vi "Logging with Helper-VIs.vi"() -> ()   [LabVIEW 2016]
doc: "HSE-Logger example using the helper VIs."
uses:
  HSE-Logger/LogLevel.ctl
  HSE-Logger/Formatter/HSE_v2_Formatter/HSE_v2_Formatter.lvclass
  C:/_work/hampel-soft/open-source/hse-logger/Source/HSE-Logger/Formatter/Formatter.lvclass
  HSE-Logger/Handler/UserEventHandler/UserEventHandler.lvclass
  C:/_work/hampel-soft/open-source/hse-logger/Source/HSE-Logger/Handler/Handler.lvclass
  HSE-Logger/Handler/FileHandler/FileHandler.lvclass
  HSE-Logger/hse-logger.lvlib
  HSE-Logger/Formatter/JSONLFormatter/JSONLFormatter.lvclass
  HSE-Logger/Formatter/Formatter.lvclass
panel:
  out "Displays log messages =>":string
  in  "btn_Log":bool
  in  "Level of Log Message":T1(ring)
  in  "Log Error":errorcluster
  in  "Log Message":string
  out "Display User Event Logs":string
  in  "btn_Exit":bool
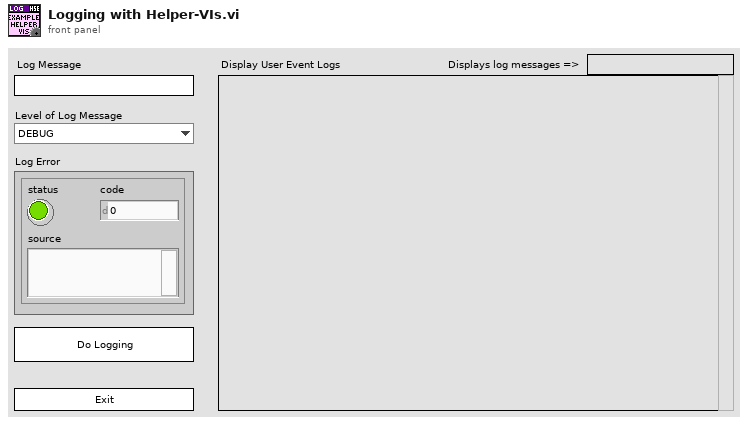
[diagram p1: front panel]
types:
  T1 = enum16{"DEBUG", "INFO", "WARNING", "ERROR", "CRITICAL"}
  T2 = typedef "hse-logger.lvlib/LogLevel.ctl" = enum16{"DEBUG", "INFO", "WARNING", "ERROR", "CRITICAL"}
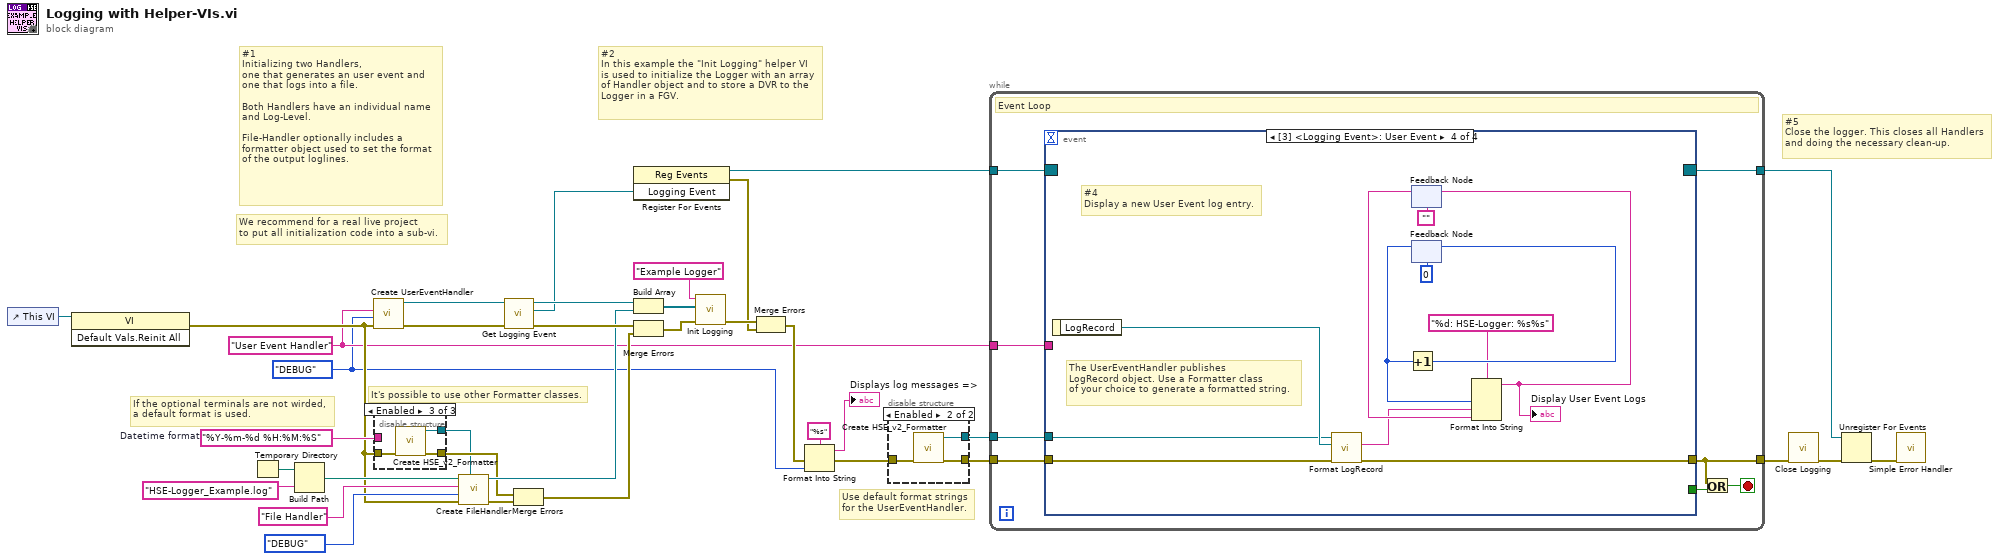
[diagram p0: block diagram]
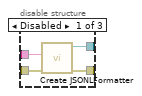
[diagram p2: hidden frame]
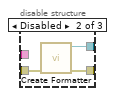
[diagram p3: hidden frame]
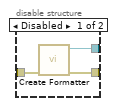
[diagram p4: hidden frame]
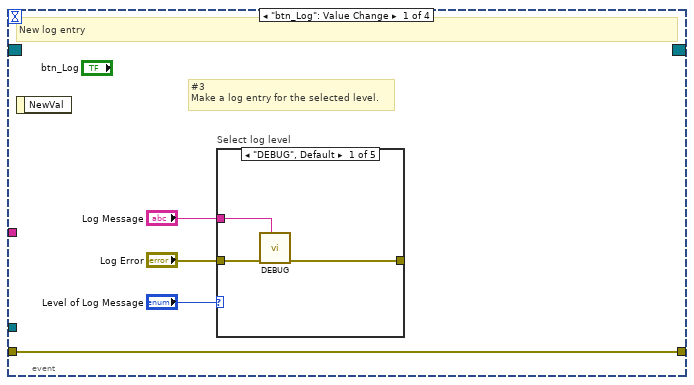
[diagram p5: hidden frame]
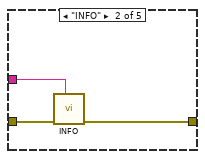
[diagram p6: hidden frame]
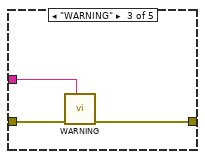
[diagram p7: hidden frame]
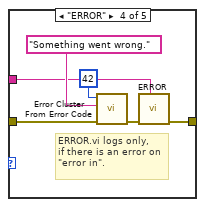
[diagram p8: hidden frame]
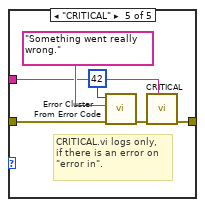
[diagram p9: hidden frame]
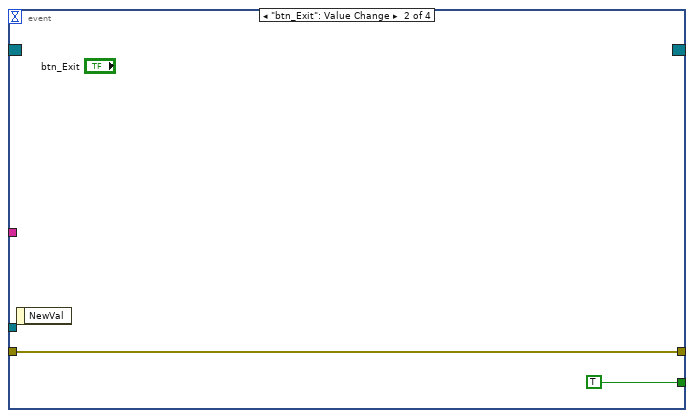
[diagram p10: hidden frame]
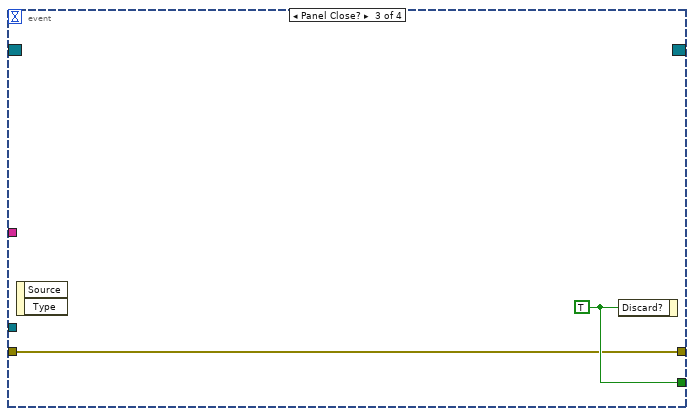
[diagram p11: hidden frame]
diagram:
  w9 = "%Y-%m-%d %H:%M:%S"  # Datetime format
  w1 = LogLevel."DEBUG" ("Level")
  w2 = "User Event Handler" ("Name")
  # "Use default format strings\nfor the UserEventHandler."
  # "If the optional terminals are not wirded,\na default format is used."
  # "It's possible to use other Formatter classes."
  # "We recommend for a real live project\nto put all initialization code into a sub-vi."
  # "#5\nClose the logger. This closes all Handlers\nand doing the necessary clean-up."
  # "#2\nIn this example the \"Init Logging\" helper VI \nis used to initialize the Logger with an array\nof Handler object and to store a DVR to the\nLogger in a FGV."
  # "#1\nInitializing two Handlers,\none that generates an user event and\none that logs into a file.\n\nBoth Handlers have an individual name\nand Log-Level.\n\nFile-Handler optionally includes a\nformatter object used to set the format\nof the output loglines."
  n1 = control-ref of="This VI"() -> (w25:refnum<vi>)
  n2 = invoke class="VI" method="Default Vals.Reinit All"(reference=w25) -> (error out=w8:errorcluster)  [unwired: 2 in, 2 out]
  n3 = Temporary Directory() -> (w24:path)
  n4 = Build Path(base path=w24, name or relative path="HSE-Logger_Example.log") -> (appended path=w14:path)
  n5 = call "Create UserEventHandler.vi"("error in"=w8, "Level"=w1, "Name"=w2) -> ("error out"=w17:errorcluster, "UserEventHandler out"=w13:refnum<class "UserEventHandler.lvclass">)  [unwired: 7 in]
  n6 = disable-structure shown="Enabled" {
    disable-tunnel: w9 -> [w40 _ _]
    disable-tunnel: w8 -> [w39 w43 w46]
    disable-tunnel: [w38 w42 w45] -> w7
    disable-tunnel: [w37 w41 w44] -> w3
    frame Disabled {
      n7 = call "Create JSONLFormatter.vi"("error in"=w39, "Datetime format"=w40) -> ("error out"=w38:errorcluster, "JSONLFormatter out"=w37:refnum<class "JSONLFormatter.lvclass">)  [unwired: 8 in]
    }
    frame Disabled {
      n8 = call "Create Formatter.vi"("error in"=w43) -> ("error out"=w42:errorcluster, "Formatter out"=w41:refnum<class "Formatter.lvclass">)  [unwired: 9 in]
    }
    frame Enabled {
      n9 = call "Create HSE_v2_Formatter.vi"("error in"=w46) -> ("error out"=w45:errorcluster, "HSE_v2_Formatter out"=w44:refnum<class "HSE_v2_Formatter.lvclass">)  [unwired: 9 in]
    }
  }
  n10 = call "Create FileHandler.vi"("Formatter.lvclass"=w3, "error in"=w8, "Level"=LogLevel."DEBUG", "Name"="File Handler", "Filepath"=w14) -> ("error out"=w12:errorcluster, "FileHandler out"=w10:refnum<class "FileHandler.lvclass">)  [unwired: 5 in]
  n11 = call-dynamic "Get Logging Event.vi"("error in"=w17, "UserEventHandler in"=w13) -> ("error out"=w33:errorcluster, "Logging Event"=w31:refnum<user-event>, "UserEventHandler out"=w32:refnum<class "UserEventHandler.lvclass">)  [unwired: 7 in]
  n12 = Merge Errors(w7, w12) -> (w11:errorcluster)
  n13 = register-events(w31) -> (reference out=w30:refnum<event-registration>, error out=w28:errorcluster)  [unwired: 2 in]
  n14 = Build Array(w32, w10) -> (w35:refnum<class "Handler.lvclass">[])
  n15 = Merge Errors(w33, w11) -> (w34:errorcluster)
  n16 = call "Init Logging.vi"("error in"=w34, "Handlers"=w35, "Name"="Example Logger") -> ("error out"=w29:errorcluster)  [unwired: 8 in]
  n17 = Merge Errors(w29, w28) -> (w21:errorcluster)
  n18 = Format Into String(format string="%s", error in=w21, w1) -> (resulting string=→"Displays log messages =>":string, error out=w6:errorcluster)  [unwired: 1 in]
  n19 = disable-structure shown="Enabled" {
    disable-tunnel: w6 -> [w49 w52]
    disable-tunnel: [w48 w51] -> w5
    disable-tunnel: [w47 w50] -> w4
    frame Disabled {
      n20 = call "Create Formatter.vi"("error in"=w49) -> ("error out"=w48:errorcluster, "Formatter out"=w47:refnum<class "Formatter.lvclass">)  [unwired: 9 in]
    }
    frame Enabled {
      n21 = call "Create HSE_v2_Formatter.vi"("error in"=w52) -> ("error out"=w51:errorcluster, "HSE_v2_Formatter out"=w50:refnum<class "HSE_v2_Formatter.lvclass">)  [unwired: 9 in]
    }
  }
  n22 = while {
    tunnel: w30 -> [w60]
    tunnel: w5 -> [w59]
    tunnel: [w57] -> w26
    tunnel: [w55] -> w18
    tunnel: w2 -> [w54]
    tunnel: w4 -> [w53]
    stop <- w56 stop-if-true
    # "Event Loop"
    n23 = event shown="[3] <Logging Event>: User Event" {
      selector: w60 -> [_ _ _ _]
      dyn-events: [_ _ _ _] -> w57
      timeout: _ -> [_ _ _ _]
      tunnel: w59 -> [w62 w86 w88 w90]
      tunnel: [_ TRUE w89 _] -> w58
      tunnel: [w62 w86 w88 w94] -> w55
      tunnel: w54 -> [_ _ _ _]
      tunnel: w53 -> [_ _ _ w91]
      event "btn_Log": Value Change {
        # "#3\nMake a log entry for the selected level."
        # "New log entry"
        n24 = event-data() -> ()  [unwired: 1 in, 1 out]
        n25 = case "Select log level" shown="\"DEBUG\", Default" "Level of Log Message" {
          tunnel: "Log Error" -> [w67 w70 w73 w79 w82]
          tunnel: [w66 w69 w72 w78 w85] -> _
          tunnel: "Log Message" -> [w65 w68 w71 w74 w80]
          frame "DEBUG", Default {
            n26 = call "DEBUG.vi"("Message"=w65, "error in"=w67) -> ("error out"=w66:errorcluster)  [unwired: 9 in]
          }
          frame "INFO" {
            n27 = call "INFO.vi"("Message"=w68, "error in"=w70) -> ("error out"=w69:errorcluster)  [unwired: 9 in]
          }
          frame "WARNING" {
            n28 = call "WARNING.vi"("Message"=w71, "error in"=w73) -> ("error out"=w72:errorcluster)  [unwired: 9 in]
          }
          frame "ERROR" {
            # "ERROR.vi logs only,\nif there is an error on\n\"error in\"."
            n29 = call <vilib>:"Error Cluster From Error Code.vi"("error in (no error)"=w79, "error message (\"\")"="Something went wrong." ("error message (\"\")"), "error code (0)"=42) -> ("error out"=w77:errorcluster)  [unwired: 6 in]
            n30 = call "ERROR.vi"("Message"=w74, "error in"=w77) -> ("error out"=w78:errorcluster)  [unwired: 9 in]
          }
          frame "CRITICAL" {
            # "CRITICAL.vi logs only,\nif there is an error on\n\"error in\"."
            n31 = call <vilib>:"Error Cluster From Error Code.vi"("error in (no error)"=w82, "error message (\"\")"="Something went really wrong." ("error message (\"\")"), "error code (0)"=42) -> ("error out"=w81:errorcluster)  [unwired: 6 in]
            n32 = call "CRITICAL.vi"("Message"=w80, "error in"=w81) -> ("error out"=w85:errorcluster)  [unwired: 9 in]
          }
        }
      }
      event "btn_Exit": Value Change {
        n33 = event-data() -> ()  [unwired: 1 in, 1 out]
      }
      event Panel Close? {
        w89 = TRUE ("Discard?")
        n34 = event-data() -> ()  [unwired: 1 in, 2 out]
        n35 = event-data("Discard?"=w89) -> ()  [unwired: 1 in, 1 out]
      }
      event User Event {
        # "The UserEventHandler publishes\nLogRecord object. Use a Formatter class\nof your choice to generate a formatted string."
        # "#4\nDisplay a new User Event log entry."
        n36 = event-data() -> ("LogRecord"=w93:refnum<class "LogRecord.lvclass">)  [unwired: 1 in]
        n37 = call-dynamic "Format LogRecord.vi"("error in"=w90, "LogRecord"=w93, "HSE_v2_Formatter in"=w91) -> ("error out"=w94:errorcluster, "LogLine"=w92:string)  [unwired: 7 in]
        n38 = feedback #1("") -> (w96:string)
        n39 = feedback #2(0) -> (w97:i32)
        n40 = Increment(x=w97) -> (x+1=w99:i32)
        n41 = feedback-in #2(w99) -> ()
        n42 = Format Into String(format string="%d: HSE-Logger: %s%s", w97, w92, w96) -> (resulting string=w98:string)  [unwired: 2 in, 1 out]
        "Display User Event Logs" <- w98
        n43 = feedback-in #1(w98) -> ()
      }
    }
    n44 = Or(x=w55, y=w58) -> (x .or. y?=w56:bool)
  }
  n45 = call "Close Logging.vi"("error in"=w18) -> ("error out"=w27:errorcluster)  [unwired: 10 in]
  n46 = Unregister For Events(event registration refnum=w26, error in=w27) -> (error out=w19:errorcluster)
  n47 = call <vilib>:"Simple Error Handler.vi"("error in (no error)"=w19) -> ()  [unwired: 4 in, 5 out]
